vi "Arroyo LaserSource Test.vi"() -> ()   [LabVIEW 2013]
panel:
  in  "Laser On":bool
  out "Voltage":dbl format="%.3g"
  in  "Set":bool
  in  "Setpoint":dbl min=-99.0 max=250.0 step=0.01 format="%.1g"
  in  "Run":bool
  out "Current":dbl format="%.1g"
  in  "COM Port":u16=1
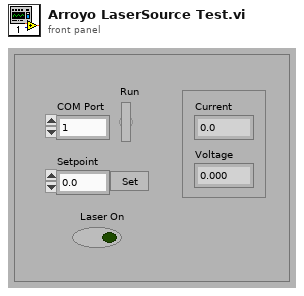
[diagram p1: front panel]
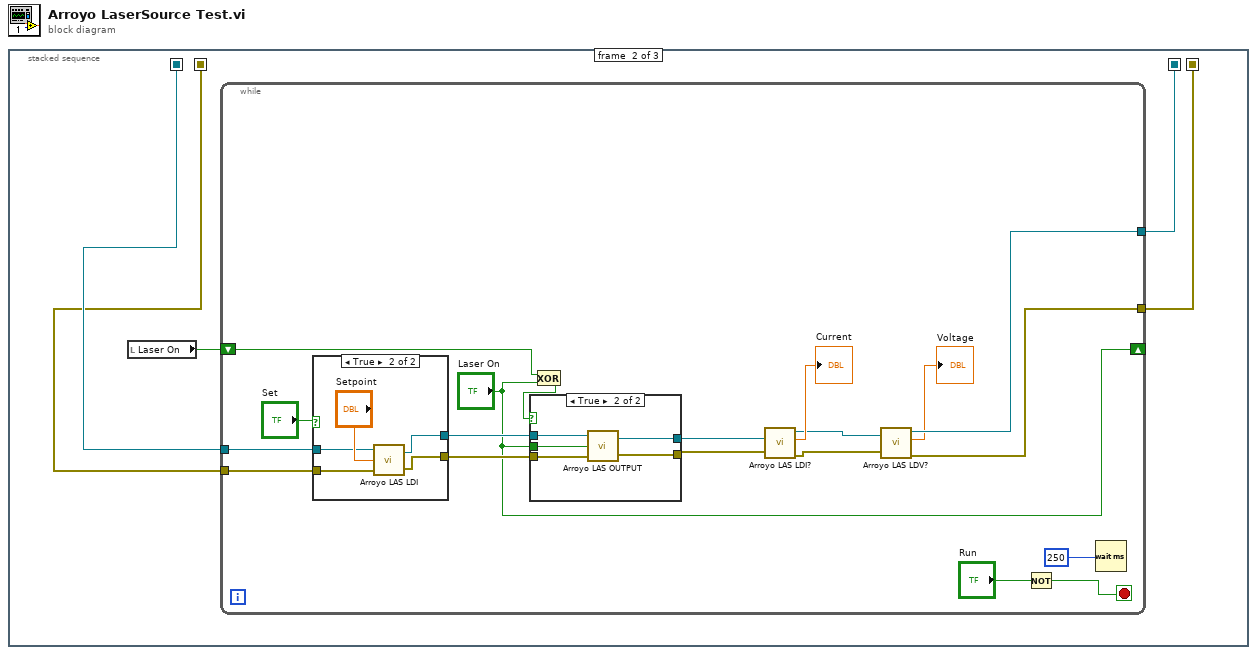
[diagram p0: block diagram]
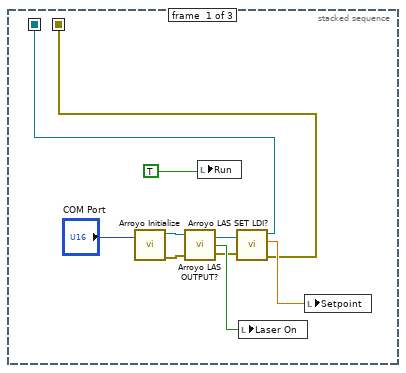
[diagram p2: hidden frame]
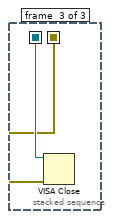
[diagram p5: hidden frame]
diagram:
  n1 = stacked-sequence {
    seq-local: [w5 _ _] -> [_ w12 _]
    seq-local: [w4 _ _] -> [_ w11 _]
    seq-local: [_ w15 _] -> [_ _ w50]
    seq-local: [_ w14 _] -> [_ _ w49]
    frame #0 {
      n2 = call "Arroyo Initialize.vi"("COM Port"="COM Port") -> ("dup VISA resource name"=w2:refnum<visa-resource-name>, "error out"=w3:errorcluster)  [unwired: 3 in]
      n3 = call "Arroyo LAS OUTPUT?.vi"("error in (no error)"=w3, "VISA resource name"=w2) -> ("error out"=w8:errorcluster, "dup VISA resource name"=w7:refnum<visa-resource-name>, "Laser Output"=w9:bool)
      n4 = local write "Run"(TRUE) -> ()
      n5 = call "Arroyo LAS SET LDI?.vi"("error in (no error)"=w8, "VISA resource name"=w7) -> ("error out"=w4:errorcluster, "Laser Current Setpoint"=w10:dbl, "dup VISA resource name"=w5:refnum<visa-resource-name>)  [unwired: 2 in]
      n6 = local write "Laser On"(w9) -> ()
      n7 = local write "Setpoint"(w10) -> ()
    }
    frame #1 {
      n8 = local read "Laser On"() -> (w13:bool)
      n9 = while {
        tunnel: [w27] -> w14
        tunnel: [w29] -> w15
        shift-right: ["Laser On"] -> _
        shift-left: w13 -> [w26]
        tunnel: w12 -> [w21]
        tunnel: w11 -> [w20]
        stop <- w31 stop-if-true
        n10 = case shown="True" "Set" {
          tunnel: [w42 w47] -> w24
          tunnel: [w43 w46] -> w23
          tunnel: w21 -> [w43 w45]
          tunnel: w20 -> [w42 w44]
          frame False {
          }
          frame True {
            n11 = call "Arroyo LAS LDI.vi"("error in (no error)"=w44, "Laser Current Setpoint"="Setpoint", "VISA resource name"=w45) -> ("error out"=w47:errorcluster, "dup VISA resource name"=w46:refnum<visa-resource-name>)
          }
        }
        n12 = Exclusive Or(1:"Laser On", 2:w26) -> (0:w25:bool)
        n13 = case shown="True" w25 {
          tunnel: "Laser On" -> [_ w41]
          tunnel: w24 -> [w35 w40]
          tunnel: w23 -> [w36 w39]
          tunnel: [w36 w38] -> w19
          tunnel: [w35 w37] -> w18
          frame False {
          }
          frame True {
            n14 = call "Arroyo LAS OUTPUT.vi"("error in (no error)"=w40, "Laser Output Enable"=w41, "VISA resource name"=w39) -> ("error out"=w37:errorcluster, "dup VISA resource name"=w38:refnum<visa-resource-name>)
          }
        }
        n15 = call "Arroyo LAS LDI?.vi"("error in (no error)"=w18, "VISA resource name"=w19) -> ("error out"=w16:errorcluster, "Laser Current"=→"Current":dbl, "dup VISA resource name"=w17:refnum<visa-resource-name>)  [unwired: 2 in]
        n16 = call "Arroyo LAS LDV?.vi"("error in (no error)"=w16, "VISA resource name"=w17) -> ("error out"=w27:errorcluster, "Laser Voltage"=→"Voltage":dbl, "dup VISA resource name"=w29:refnum<visa-resource-name>)  [unwired: 2 in]
        n17 = Not(x="Run") -> (.not. x?=w31:bool)
        n18 = Wait (ms)(milliseconds to wait=250) -> ()  [unwired: 1 out]
      }
    }
    frame #2 {
      n19 = VISA Close(VISA resource name=w50, error in (no error)=w49) -> ()  [unwired: 1 out]
    }
  }
